vi "make_path_relative.vi"(8 "error in (no error)":errorcluster, 11 "absolute path":path) -> (0 "error out":errorcluster, 3 "relative path":string)   [LabVIEW 2010]
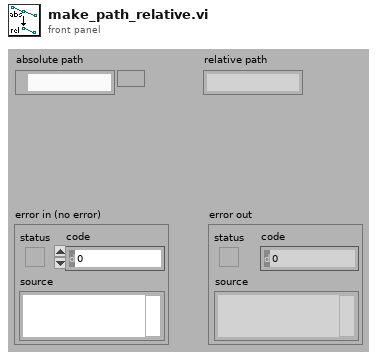
[diagram p1: front panel]
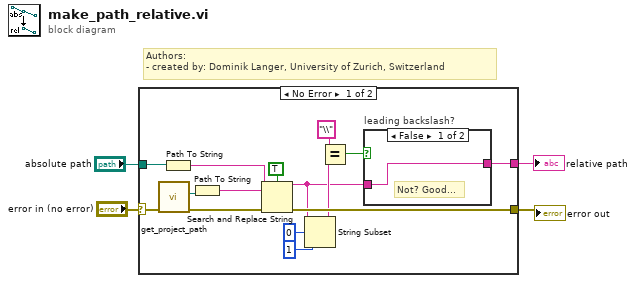
[diagram p0: block diagram]
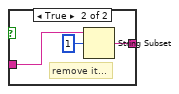
[diagram p2: hidden frame]
diagram:
  # "Authors: \n- created by: Dominik Langer, University of Zurich, Switzerland"
  n1 = case shown="No Error" "error in (no error)" {
    selector: "error in (no error)" -> [w19 w24]
    tunnel: "absolute path" -> [w17 _]
    tunnel: [w15 w24] -> w2
    tunnel: [w5 _] -> w1
    frame No Error {
      n2 = call "get_project_path.vi"("error in (no error)"=w19) -> ("error out"=w16:errorcluster, "helioscan path"=w18:path)  [unwired: 9 in]
      n3 = Path To String(path=w17) -> (string=w14:string)
      n4 = Path To String(path=w18) -> (string=w13:string)
      n5 = Search and Replace String(case sensitive?=TRUE ("ignore case? (F)"), input string=w14, search string=w13, error in=w16) -> (result string=w6:string, error out=w15:errorcluster)  [unwired: 4 in, 2 out]
      n6 = String Subset(string=w6, offset (0)=0, length (rest)=1 ("length (rest)")) -> (substring=w9:string)
      n7 = Equal?(x="\\", y=w9) -> (x = y?=w7:bool)
      n8 = case "leading backslash?" shown="False" w7 {
        tunnel: w6 -> [w20 w23]
        tunnel: [w20 w21] -> w5
        frame False {
          # "Not? Good..."
        }
        frame True {
          # "remove it..."
          n9 = String Subset(string=w23, offset (0)=1) -> (substring=w21:string)  [unwired: 1 in]
        }
      }
    }
    frame Error {
    }
  }
  "error out" <- w2
  "relative path" <- w1
